vi "Ballard XML Generator.Add Label.vi"(6 "SDI":i32, 7 "other params":string[](array[string]), 8 "label decimal":i32, 9 "name":string, 10 "id":string, 11 "string in":string) -> (3 "string out":string)   [LabVIEW 2017]
uses:
  <vilib>/Utility/error.llb/whitespace.ctl
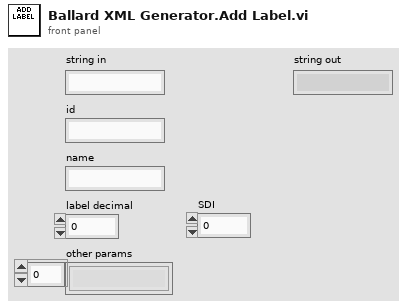
[diagram p1: front panel]
types:
  T1 = typedef "whitespace.ctl" = u16
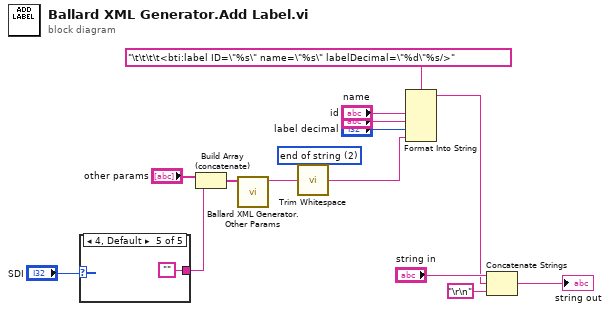
[diagram p0: block diagram]
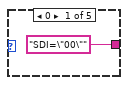
[diagram p2: hidden frame]
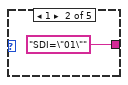
[diagram p3: hidden frame]
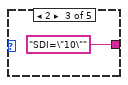
[diagram p4: hidden frame]
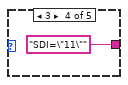
[diagram p5: hidden frame]
diagram:
  w2 = T1 2 items=["both", "start of string", "end of string"] ("location (both)")
  n1 = case shown="4, Default" "SDI" {
    tunnel: ["SDI=\"00\"" "SDI=\"01\"" "SDI=\"10\"" "SDI=\"11\"" ""] -> w4
    frame 0 {
    }
    frame 1 {
    }
    frame 2 {
    }
    frame 3 {
    }
    frame 4, Default {
    }
  }
  n2 = Build Array (concatenate)("other params", w4) -> (w5:string[])
  n3 = call "Ballard XML Generator.Other Params.vi"("other params"=w5) -> ("string"=w3:string)  [unwired: 10 in]
  n4 = call <vilib>:"Trim Whitespace.vi"("string"=w3, "location (both)"=w2) -> ("trimmed string"=w1:string)
  n5 = Format Into String(format string="\t\t\t\t<bti:label ID=\"%s\" name=\"%s\" labelDecimal=\"%d\"%s/>", "id", "name", "label decimal", w1) -> (resulting string=w7:string)  [unwired: 2 in, 1 out]
  n6 = Concatenate Strings("string in", w7, "\r\n") -> (→"string out":string)
